vi "Simple Capture Scan Counter.vi"(8 "Scan Tracker":T1) -> (0 "Scan Tracker Out":T1, 1 "To cycle?":bool, 3 "Exit?":bool)   [LabVIEW 2016]
uses:
  Simple Capture Manager Controls/Simple Capture Scan Tracker.ctl
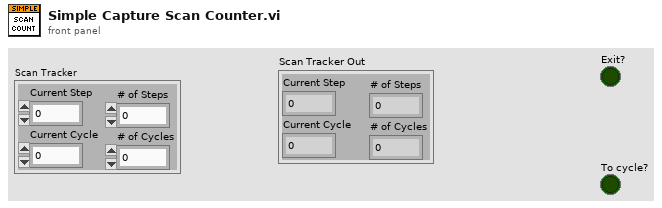
[diagram p1: front panel]
types:
  T1 = typedef "Simple Capture Scan Tracker.ctl" = cluster{"Current Step":u32, "Current Cycle":u32, "# of Cycles":u32, "# of Steps":u32}
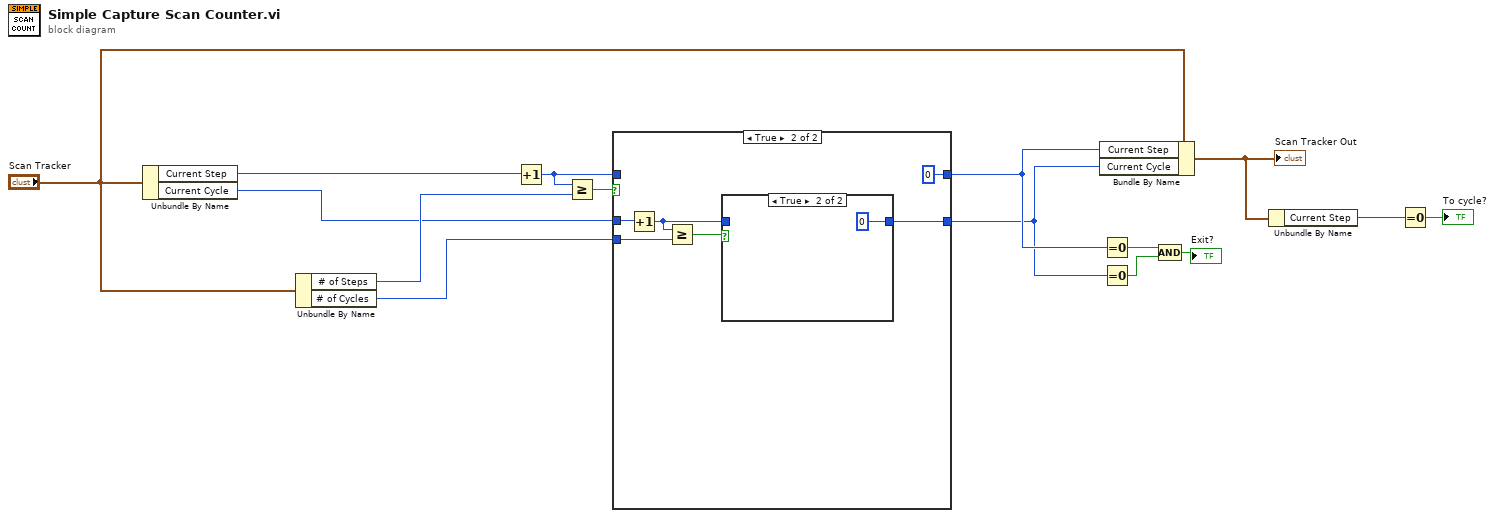
[diagram p0: block diagram]
diagram:
  n1 = Unbundle By Name("Scan Tracker") -> ("Current Step"=w15:u32, "Current Cycle"=w13:u32)
  n2 = Unbundle By Name("Scan Tracker") -> ("# of Steps"=w14:u32, "# of Cycles"=w12:u32)
  n3 = Increment(x=w15) -> (x+1=w2:u32)
  n4 = Greater Or Equal?(x=w2, y=w14) -> (x >= y?=w1:bool)
  n5 = case shown="True" w1 {
    tunnel: w2 -> [w17 _]
    tunnel: [w17 u32 0] -> w11
    tunnel: w13 -> [w16 w22]
    tunnel: w12 -> [_ w21]
    tunnel: [w16 w18] -> w10
    frame False {
    }
    frame True {
      n6 = Increment(x=w22) -> (x+1=w20:u32)
      n7 = Greater Or Equal?(x=w20, y=w21) -> (x >= y?=w19:bool)
      n8 = case shown="True" w19 {
        tunnel: w20 -> [w24 _]
        tunnel: [w24 u32 0] -> w18
        frame False {
        }
        frame True {
        }
      }
    }
  }
  n9 = Bundle By Name(cluster="Scan Tracker", "Current Step"=w11, "Current Cycle"=w10) -> (w6:T1)
  "Scan Tracker Out" <- w6
  n10 = Equal To 0?(x=w11) -> (x = 0?=w9:bool)
  n11 = Equal To 0?(x=w10) -> (x = 0?=w8:bool)
  n12 = Compound Arithmetic op=AND(w9, w8) -> (→"Exit?":bool)
  n13 = Unbundle By Name(w6) -> ("Current Step"=w5:u32)
  n14 = Equal To 0?(x=w5) -> (x = 0?=→"To cycle?":bool)
